vi "Initialize Core.vi"(8 "Error In":errorcluster, 11 "BNT_SLMsgLogger in":refnum<class "BNT_SLMsgLogger.lvclass">) -> (0 "Error Out":errorcluster, 3 "BNT_SLMsgLogger out":refnum<class "BNT_SLMsgLogger.lvclass">)   [LabVIEW 2019, in "BNT_SLMsgLogger.lvlib" / "BNT_SLMsgLogger.lvclass"]
doc: "Initialize the message logger."
uses:
  BNT_SLMsgLogger.lvclass
  BNT_SLMsgLogger.lvclass/BNT_SLMsgLogger.ctl
  <vilib>/Skyline/Configuration/Configuration AMQP_class/NI Skyline Configuration AMQP.lvclass
  <vilib>/Skyline/Configuration/Configuration HTTP_class/NI Skyline Configuration HTTP.lvclass
  <vilib>/Skyline/Message/AMQP/NI Skyline Message AMQP (Async).lvclass
  C:/Program Files (x86)/National Instruments/LabVIEW 2019/vi.lib/Skyline/Message/NI Skyline Message.lvclass
  <vilib>/Skyline/Message/HTTP Wrapper/NI Skyline Message HTTP.lvclass
  <vilib>/Skyline/Message/AMQP/NI Skyline Message AMQP (Sync).lvclass
  <vilib>/Skyline/Message/AMQP/async/Open (Async).vi
  <vilib>/Skyline/Message/HTTP Wrapper/Open (HTTP).vi
  <vilib>/Skyline/Message/AMQP/sync/Open (Sync).vi
  <vilib>/Skyline/Message/NI Skyline Message.lvclass
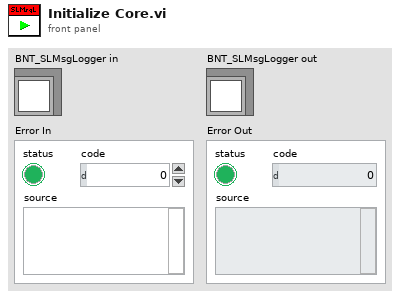
[diagram p1: front panel]
types:
  T1 = typedef "BNT_SLMsgLogger.lvlib/BNT_SLMsgLogger.lvclass/Protocol.ctl" = enum16{"AMQPSync", "AMQPAsync", "HTTP"}
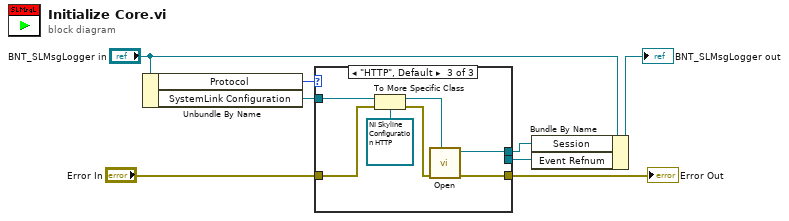
[diagram p0: block diagram]
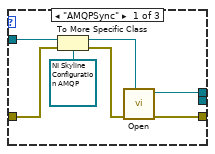
[diagram p2: hidden frame]
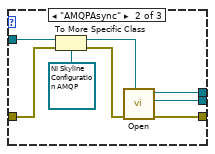
[diagram p3: hidden frame]
diagram:
  n1 = Unbundle By Name("BNT_SLMsgLogger in") -> ("Protocol"=w6:T1, "SystemLink Configuration"=w1:refnum<class "NI Skyline Configuration.lvclass">)
  n2 = case shown="\"HTTP\", Default" w6 {
    tunnel: "Error In" -> [w9 w16 w24]
    tunnel: [w15 w23 w30] -> w7
    tunnel: [w14 w22 w29] -> w2
    tunnel: [_ w21 _] -> w3
    tunnel: w1 -> [w13 w20 w28]
    frame "AMQPSync" {
      n3 = To More Specific Class(target class=refnum<class "NI Skyline Configuration AMQP.lvclass"> refnum ("configuration"), reference=w13, error in=w9) -> (specific class reference=w11:refnum<class "NI Skyline Configuration AMQP.lvclass">, error out=w10:errorcluster)
      n4 = call-poly <vilib>:"Open.vi"("configuration"=w11, "error in (no error)"=w10) -> ("error out"=w15:errorcluster, "message session"=w14:refnum<class "NI Skyline Message AMQP (Sync).lvclass">)  [unwired: 8 in]
    }
    frame "AMQPAsync" {
      n5 = To More Specific Class(target class=refnum<class "NI Skyline Configuration AMQP.lvclass"> refnum ("configuration"), reference=w20, error in=w16) -> (specific class reference=w19:refnum<class "NI Skyline Configuration AMQP.lvclass">, error out=w17:errorcluster)
      n6 = call-poly <vilib>:"Open.vi"("configuration"=w19, "error in (no error)"=w17) -> ("error out"=w23:errorcluster, "event registration refnum"=w21:refnum<event-registration>, "message session"=w22:refnum<class "NI Skyline Message AMQP (Async).lvclass">)  [unwired: 7 in]
    }
    frame "HTTP", Default {
      n7 = To More Specific Class(target class=refnum<class "NI Skyline Configuration HTTP.lvclass"> refnum ("HTTP configuration out"), reference=w28, error in=w24) -> (specific class reference=w27:refnum<class "NI Skyline Configuration HTTP.lvclass">, error out=w25:errorcluster)
      n8 = call-poly <vilib>:"Open.vi"("configuration"=w27, "error in (no error)"=w25) -> ("error out"=w30:errorcluster, "message session"=w29:refnum<class "NI Skyline Message HTTP.lvclass">)  [unwired: 8 in]
    }
  }
  "Error Out" <- w7
  n9 = Bundle By Name(cluster="BNT_SLMsgLogger in", "Session"=w2, "Event Refnum"=w3) -> (→"BNT_SLMsgLogger out":refnum<class "BNT_SLMsgLogger.lvclass">)
